vi "Transfer Group Count.vi"   [LabVIEW 2017, in "DSF Core.lvlib" / "Configuration Session.lvclass"]
uses:
  Configuration Session.lvclass
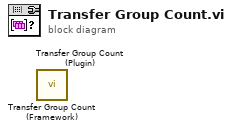
[diagram p0: block diagram]
diagram:
  n1 = call "Transfer Group Count (Framework).vi"() -> ()  [unwired: 9 in, 3 out]
  n2 = call "Transfer Group Count (Plugin).vi"() -> ()  [unwired: 9 in, 3 out]
